vi "Restore Tree Collapsed State.vi"(0 "TreeControl in":refnum<vi>, 1 "Array":string[](array[string]), 5 "error in (no error)":errorcluster) -> (14 "TreeControl out":refnum<vi>, 19 "error out":errorcluster)   [LabVIEW 2023, in "Message Maker.lvclass"]
uses:
  Message Maker.lvclass
  Message Maker.lvclass/Message Maker.ctl
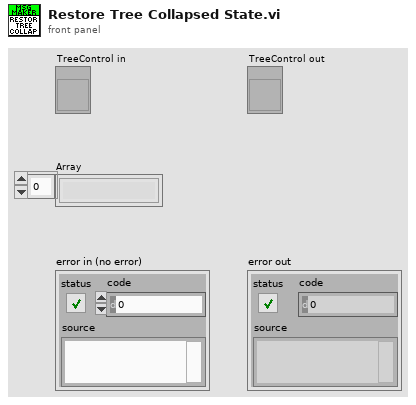
[diagram p1: front panel]
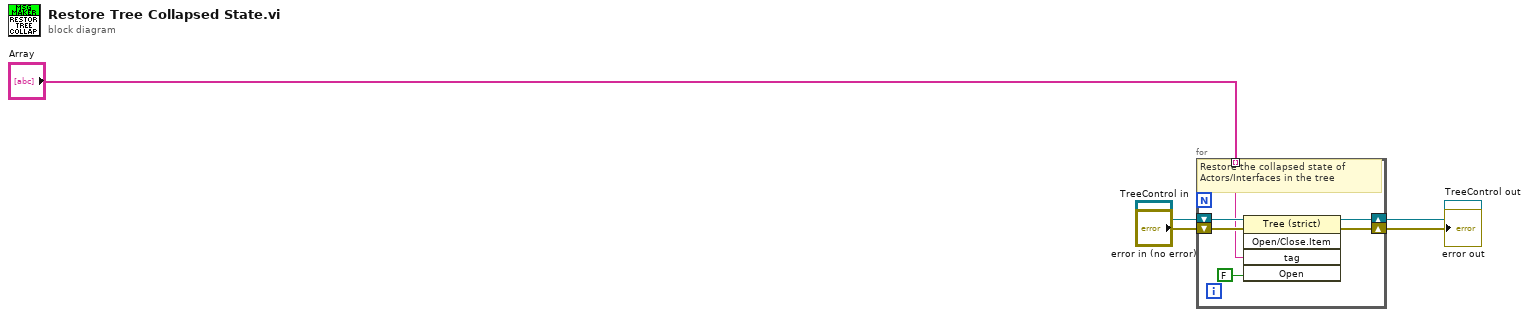
[diagram p0: block diagram]
diagram:
  n1 = for {
    shift-right: [w9] -> w3
    shift-left: "TreeControl in" -> [w11]
    shift-right: [w8] -> w4
    shift-left: "error in (no error)" -> [w10]
    tunnel: "Array" -> [w7] mode=indexing
    # "Restore the collapsed state of Actors/Interfaces in the tree"
    n2 = invoke class="Tree (strict)" method="Open/Close.Item"(reference=w11, error in=w10, "tag"=w7, "Open"=FALSE ("Open?")) -> (reference out=w9:refnum<vi>, error out=w8:errorcluster)  [unwired: 1 in, 3 out]
  }
  "error out" <- w4
  "TreeControl out" <- w3
